vi "Process.vi"(11 "Process In":refnum<class "Process.lvclass">) -> ()   [LabVIEW 2020, in "Process.lvclass"]
uses:
  Process.lvclass
  C:/git/astemes-triarc-framework/source/Framework/Logging/Logging.lvclass
  Process.lvclass/Process.ctl
  Logging/Log Warning.vi
  Logging/Log Error.vi
  Logging/Log Debug.vi
  <vilib>/AdvancedString/1D String Array to Delimited String.vi
  <vilib>/Utility/High Resolution Relative Seconds.vi
  <vilib>/Utility/error.llb/Error Cluster From Error Code.vi
  Public/Read Name.vi
  Logging/Logging.lvclass
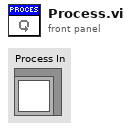
[diagram p1: front panel]
types:
  T1 = enum16{"Send", "Receive", "Request", "Response", "Broadcast"}
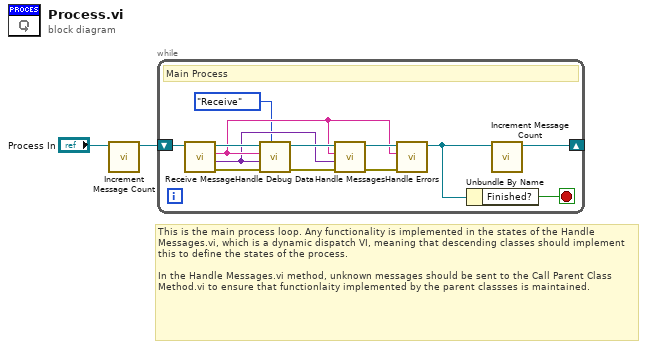
[diagram p0: block diagram]
diagram:
  # "This is the main process loop. Any functionality is implemented in the states of the Handle Messages.vi, which is a dynamic dispatch VI, meaning that descending classes should implement this to define the states of the process.\n\nIn the Handle Messages.vi method, unknown messages should be sent to the Call Parent Class Method.vi to ensure that functionlaity implemented by the parent classses is maintained."
  n1 = call "Increment Message Count.vi"("Process In"="Process In") -> ("Process Out"=w1:refnum<class "Process.lvclass">)  [unwired: 10 in]
  n2 = while {
    shift-right: [w4] -> _
    shift-left: w1 -> [w15]
    stop <- w5 stop-if-true
    # "Main Process"
    n3 = call "Receive Message.vi"("Process In"=w15) -> ("error out"=w13:errorcluster, "Message Data"=w7:variant, "Message"=w8:string, "Process Out"=w14:refnum<class "Process.lvclass">)  [unwired: 7 in]
    n4 = call "Handle Debug Data.vi"("Action"=T1."Receive", "error in (no error)"=w13, "Message Data"=w7, "Message"=w8, "Process In"=w14) -> ("error out"=w11:errorcluster, "Process Out"=w12:refnum<class "Process.lvclass">)  [unwired: 5 in]
    n5 = call-dynamic "Handle Messages.vi"("error in (no error)"=w11, "Message Data"=w7, "Message"=w8, "Process In"=w12) -> ("error out"=w9:errorcluster, "Process Out"=w10:refnum<class "Process.lvclass">)  [unwired: 6 in]
    n6 = call-dynamic "Handle Errors.vi"("error in (no error)"=w9, "Location"=w8, "Process In"=w10) -> ("Process Out"=w6:refnum<class "Process.lvclass">)  [unwired: 7 in, 1 out]
    n7 = Unbundle By Name(w6) -> ("Finished?"=w5:bool)
    n8 = call "Increment Message Count.vi"("Process In"=w6) -> ("Process Out"=w4:refnum<class "Process.lvclass">)  [unwired: 10 in]
  }
